vi "Read Power Measurement.vi"(7 "Detector Type (RMS)":i32(ring) items=["RMS", "Minimum", "Maximum"], 8 "error in (no error)":errorcluster, 9 "Result Type (Current)":i32(ring) items=["Current", "Average", "Peak"], 10 "Instance (1)":i32=1 format="%.0g", 11 "VISA resource name":refnum<visa-resource-name>) -> (0 "error out":errorcluster, 1 "Power":dbl[](array[numeric]) format="%^.3e", 2 "Reliability":i32, 3 "VISA resource name out":refnum<visa-resource-name>)   [LabVIEW 2020, in "Rohde&Schwarz CMXP GPRF.lvlib"]
doc: "Starts a new single shot measurement and returns the results.\n\nAttributes:\nRSCMXPGPRF_ATTR_READ_POWER_MEASUREMENT_MINIMUM_CURRENT\nRSCMXPGPRF_ATTR_READ_POWER_MEASUREMENT_MAXIMUM_CURRENT\nRSCMXPGPRF_ATTR_READ_POWER_MEASUREMENT_POWER_CURRENT\nRSCMXPGPRF_ATTR_READ_POWER_MEASUREMENT_POWER_AVERAGE\nRSCMXPGPRF_ATTR_READ_POWER_MEASUREMENT_MINIMUM_PEAK\nRSCMXPGPRF_ATTR_READ_POWER_MEASUREMENT_MAXIMUM_PEAK\n\nRemote-control commands:\nREAD:GPRF:MEAS<i>:POWer:MINimum:CURRent?\nREAD:GPRF:MEAS<i>:POWer:MAXimum:CURRent?\nREAD:GPRF:MEAS<i>:POWer:CURRent?\nREAD:GPRF:MEAS<i>:POWer:AVERage?\nREAD:GPRF:MEAS<i>:POWer:PEAK:MINimum?\nREAD:GPRF:MEAS<i>:POWer:PEAK:MAXimum?"
uses:
  <instrlib>/Rohde&Schwarz CMXP GPRF/Rohde&Schwarz CMXP GPRF.lvlib
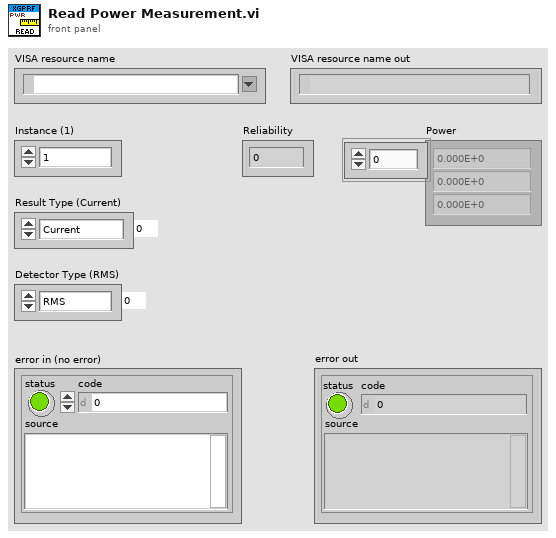
[diagram p1: front panel]
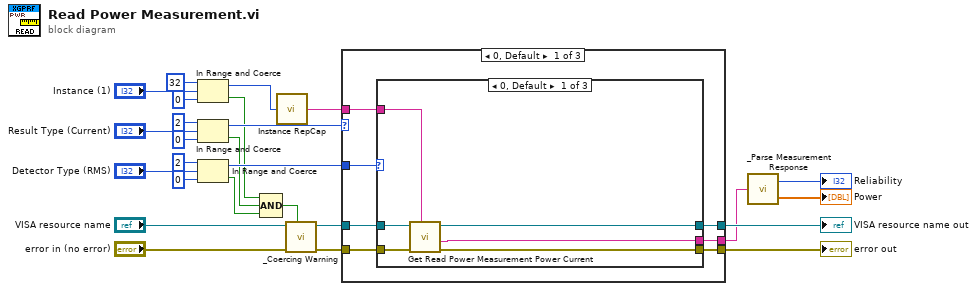
[diagram p0: block diagram]
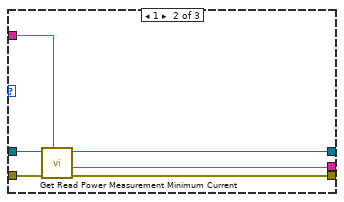
[diagram p2: hidden frame]
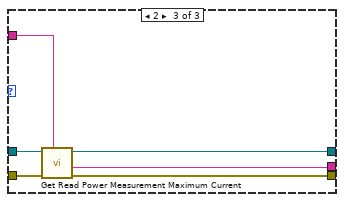
[diagram p3: hidden frame]
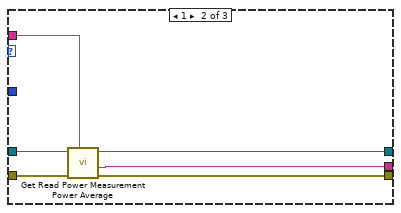
[diagram p4: hidden frame]
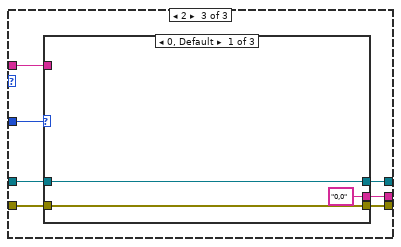
[diagram p5: hidden frame]
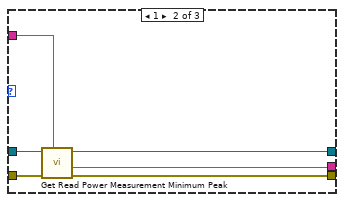
[diagram p6: hidden frame]
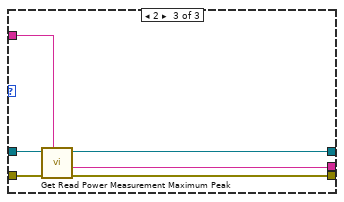
[diagram p7: hidden frame]
diagram:
  n1 = In Range and Coerce(upper limit=32, x="Instance (1)", lower limit=0) -> (coerced(x)=w5:i32, In Range?=w2:bool)
  n2 = In Range and Coerce(upper limit=2, x="Result Type (Current)", lower limit=0) -> (coerced(x)=w14:i32, In Range?=w3:bool)
  n3 = In Range and Coerce(upper limit=2, x="Detector Type (RMS)", lower limit=0) -> (coerced(x)=w9:i32, In Range?=w4:bool)
  n4 = Compound Arithmetic op=AND(w2, w3, w4) -> (w22:bool)
  n5 = call <instrlib>:"Instance RepCap.vi"("Instance in"=w5) -> ("Instance out"=w6:string)
  n6 = call <instrlib>:"_Coercing Warning.vi"("In Range?"=w22, "error in (no error)"="error in (no error)", "VISA resource name"="VISA resource name") -> ("error out"=w13:errorcluster, "VISA resource name out"=w12:refnum<visa-resource-name>)  [unwired: 7 in]
  n7 = case shown="0, Default" w14 {
    tunnel: w13 -> [w33 w57 w64]
    tunnel: w12 -> [w32 w56 w63]
    tunnel: [w31 w55 w62] -> w11
    tunnel: [w30 w54 w61] -> w10
    tunnel: w9 -> [w29 _ w60]
    tunnel: [w28 w53 w59] -> w1
    tunnel: w6 -> [w27 w52 w58]
    frame 0, Default {
      n8 = case shown="0, Default" w29 {
        tunnel: w33 -> [w39 w45 w51]
        tunnel: w32 -> [w38 w44 w50]
        tunnel: [w37 w43 w49] -> w31
        tunnel: [w36 w42 w48] -> w30
        tunnel: [w35 w41 w47] -> w28
        tunnel: w27 -> [w34 w40 w46]
        frame 0, Default {
          n9 = call "Get Read Power Measurement Power Current"("Repeated Capabilities"=w34, "error in (no error)"=w39, "instrument handle"=w38) -> ("error out"=w37:errorcluster, "Read Power Measurement Power Current"=w35:string, "instrument handle out"=w36:refnum<visa-resource-name>)  [unwired: 6 in]
        }
        frame 1 {
          n10 = call "Get Read Power Measurement Minimum Current"("Repeated Capabilities"=w40, "error in (no error)"=w45, "instrument handle"=w44) -> ("error out"=w43:errorcluster, "Read Power Measurement Minimum Current"=w41:string, "instrument handle out"=w42:refnum<visa-resource-name>)  [unwired: 6 in]
        }
        frame 2 {
          n11 = call "Get Read Power Measurement Maximum Current"("Repeated Capabilities"=w46, "error in (no error)"=w51, "instrument handle"=w50) -> ("error out"=w49:errorcluster, "Read Power Measurement Maximum Current"=w47:string, "instrument handle out"=w48:refnum<visa-resource-name>)  [unwired: 6 in]
        }
      }
    }
    frame 1 {
      n12 = call "Get Read Power Measurement Power Average"("Repeated Capabilities"=w52, "error in (no error)"=w57, "instrument handle"=w56) -> ("error out"=w55:errorcluster, "Read Power Measurement Power Average"=w53:string, "instrument handle out"=w54:refnum<visa-resource-name>)  [unwired: 6 in]
    }
    frame 2 {
      n13 = case shown="0, Default" w60 {
        tunnel: w64 -> [w67 w73 w79]
        tunnel: w63 -> [w66 w72 w78]
        tunnel: [w67 w71 w77] -> w62
        tunnel: [w66 w70 w76] -> w61
        tunnel: ["0,0" ("Read Power Measurement Maximum Current") w69 w75] -> w59
        tunnel: w58 -> [_ w68 w74]
        frame 0, Default {
        }
        frame 1 {
          n14 = call "Get Read Power Measurement Minimum Peak"("Repeated Capabilities"=w68, "error in (no error)"=w73, "instrument handle"=w72) -> ("error out"=w71:errorcluster, "Read Power Measurement Minimum Peak"=w69:string, "instrument handle out"=w70:refnum<visa-resource-name>)  [unwired: 6 in]
        }
        frame 2 {
          n15 = call "Get Read Power Measurement Maximum Peak"("Repeated Capabilities"=w74, "error in (no error)"=w79, "instrument handle"=w78) -> ("error out"=w77:errorcluster, "Read Power Measurement Maximum Peak"=w75:string, "instrument handle out"=w76:refnum<visa-resource-name>)  [unwired: 6 in]
        }
      }
    }
  }
  "error out" <- w11
  "VISA resource name out" <- w10
  n16 = call <instrlib>:"_Parse Measurement Response.vi"("String In"=w1) -> ("Reliability"=→"Reliability":i32, "Data"=→"Power":dbl[])
